vi "Release.vi"(8 "error in (no error)":errorcluster, 11 "Report in":refnum<class "Report.lvclass">) -> (0 "error out":errorcluster)   [LabVIEW 2020, in "TSnax.lvlib" / "Report.lvclass"]
uses:
  Report.lvclass
  Report.lvclass/Report.ctl
  PropertyObject/PropertyObject.lvclass
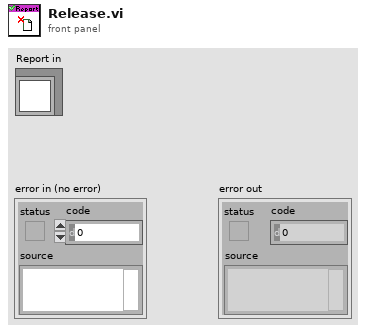
[diagram p1: front panel]
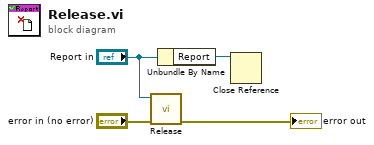
[diagram p0: block diagram]
diagram:
  n1 = call-parent "Release.vi"("error in (no error)"="error in (no error)", "PropertyObject in"="Report in") -> ("error out"=→"error out":errorcluster)  [unwired: 9 in]
  n2 = Unbundle By Name("Report in") -> ("Report"=w2:refnum<k7>)
  n3 = Close Reference(reference=w2) -> ()  [unwired: 1 in, 1 out]
